vi "Choreo_SwerveSample_Flipped.vi"(11 "ChoreoSwerveSample":T1) -> (3 "FlippedSwerveSample":T1)   [LabVIEW 2019, in "ChoreoLib.lvlib"]
doc: "Returns this sample, mirrored across the field midline.\n\nInputs:\n -- ChoreoSwerveSample - cluster - Swerve sample.\n \nOutputs: \n -- FlippedSwerveSample - cluster - This sample, mirrored across the field midline."
uses:
  ChoreoLib.lvlib
  TypeDef/ChoreoSwerveSample.ctl
  Choreo_Choreo_Globals.vi
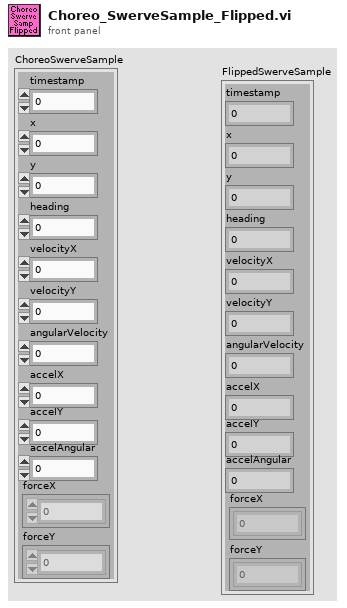
[diagram p1: front panel]
types:
  T1 = typedef "ChoreoLib.lvlib/ChoreoSwerveSample.ctl" = cluster{"timestamp":dbl, "x":dbl, "y":dbl, "heading":dbl, "velocityX":dbl, "velocityY":dbl, "angularVelocity":dbl, "accelX":dbl, "accelY":dbl, "accelAngular":dbl, "forceX":dbl[], "forceY":dbl[]}
  T2 = typedef "ChoreoLib.lvlib/Choreo_Util_AllianceFlipType.ctl" = enum16{"MIRRORED", "ROTATE_AROUND"}
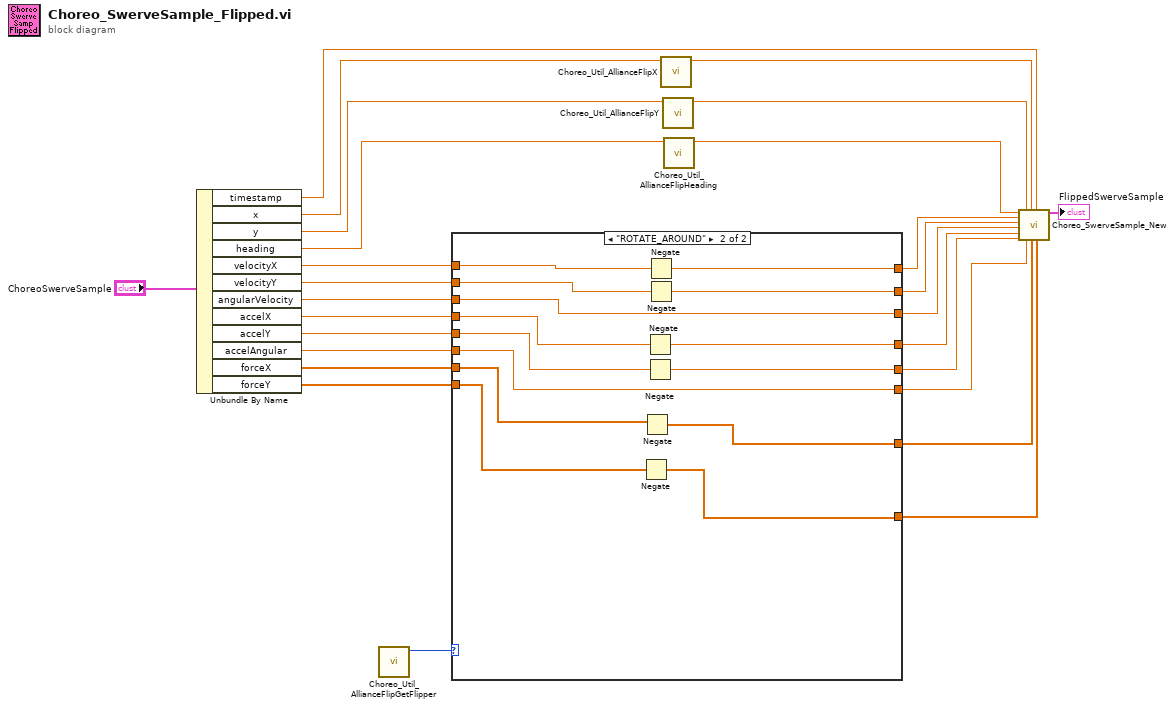
[diagram p0: block diagram]
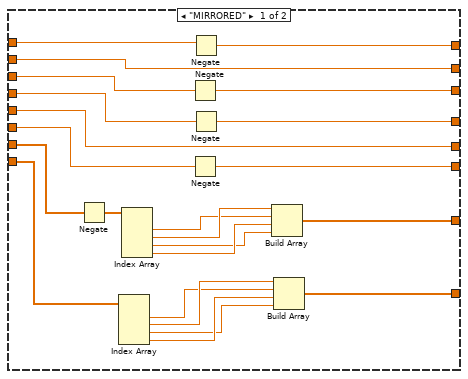
[diagram p2: hidden frame]
diagram:
  n1 = Unbundle By Name("ChoreoSwerveSample") -> ("timestamp"=w24:dbl, "x"=w21:dbl, "y"=w22:dbl, "heading"=w23:dbl, "velocityX"=w17:dbl, "velocityY"=w16:dbl, "angularVelocity"=w15:dbl, "accelX"=w14:dbl, "accelY"=w13:dbl, "accelAngular"=w12:dbl, "forceX"=w11:dbl[], "forceY"=w10:dbl[])
  n2 = call "Choreo_Util_AllianceFlipGetFlipper.vi"() -> ("Flipper"=w26:T2)  [unwired: 11 in]
  n3 = case shown="\"ROTATE_AROUND\"" w26 {
    tunnel: w17 -> [w49 w63]
    tunnel: [w48 w60] -> w8
    tunnel: w16 -> [w48 w61]
    tunnel: w15 -> [w47 w59]
    tunnel: w14 -> [w46 w58]
    tunnel: [w45 w56] -> w5
    tunnel: w13 -> [w45 w55]
    tunnel: w12 -> [w44 w54]
    tunnel: w11 -> [w42 w53]
    tunnel: w10 -> [w43 w52]
    tunnel: [w32 w62] -> w9
    tunnel: [w31 w59] -> w7
    tunnel: [w30 w57] -> w6
    tunnel: [w29 w54] -> w4
    tunnel: [w28 w51] -> w3
    tunnel: [w27 w50] -> w2
    frame "MIRRORED" {
      n4 = Negate(x=w42) -> (-x=w41:dbl[])
      n5 = Index Array(array=w43) -> (element #1=w35:dbl, element #2=w36:dbl, element #3=w33:dbl, element #4=w34:dbl)  [unwired: 4 in]
      n6 = Index Array(array=w41) -> (element #1=w39:dbl, element #2=w40:dbl, element #3=w37:dbl, element #4=w38:dbl)  [unwired: 4 in]
      n7 = Negate(x=w47) -> (-x=w31:dbl)
      n8 = Negate(x=w44) -> (-x=w29:dbl)
      n9 = Negate(x=w49) -> (-x=w32:dbl)
      n10 = Negate(x=w46) -> (-x=w30:dbl)
      n11 = Build Array(w40, w39, w38, w37) -> (w28:dbl[])
      n12 = Build Array(w36, w35, w34, w33) -> (w27:dbl[])
    }
    frame "ROTATE_AROUND" {
      n13 = Negate(x=w52) -> (-x=w50:dbl[])
      n14 = Negate(x=w53) -> (-x=w51:dbl[])
      n15 = Negate(x=w58) -> (-x=w57:dbl)
      n16 = Negate(x=w55) -> (-x=w56:dbl)
      n17 = Negate(x=w63) -> (-x=w62:dbl)
      n18 = Negate(x=w61) -> (-x=w60:dbl)
    }
  }
  n19 = call "Choreo_Util_AllianceFlipX.vi"("X"=w21) -> ("FlippedX"=w20:dbl)  [unwired: 10 in]
  n20 = call "Choreo_Util_AllianceFlipY.vi"("Y"=w22) -> ("FlippedY"=w19:dbl)  [unwired: 10 in]
  n21 = call "Choreo_Util_AllianceFlipHeading.vi"("heading"=w23) -> ("FlippedHeading"=w18:dbl)  [unwired: 10 in]
  n22 = call "Choreo_SwerveSample_New.vi"("heading"=w18, "velocityX"=w9, "velocityY"=w8, "angularVelocity"=w7, "accelX"=w6, "accelY"=w5, "y"=w19, "accelAngular"=w4, "x"=w20, "forceX"=w3, "timestamp"=w24, "forceY"=w2) -> ("ChoreoSwerveSample"=→"FlippedSwerveSample":T1)  [unwired: 7 in]
